vi "PUT File.vi"(6 "timeout (10000)":i32=10000, 7 "output file":path=path "", 8 "error in (no error)":errorcluster, 9 "file":path, 10 "url":string, 11 "HTTP Client Advanced in":refnum<class "HTTP Client Advanced.lvclass">) -> (0 "error out":errorcluster, 1 "body":string, 2 "headers":string, 3 "HTTP Client Advanced out":refnum<class "HTTP Client Advanced.lvclass">)   [LabVIEW 2021, in "HTTP Client Advanced.lvclass"]
uses:
  HTTP Client Advanced.lvclass
  HTTP Client Advanced.lvclass/HTTP Client Advanced.ctl
  <vilib>/NI/Advanced HTTP Client/Session.lvclass
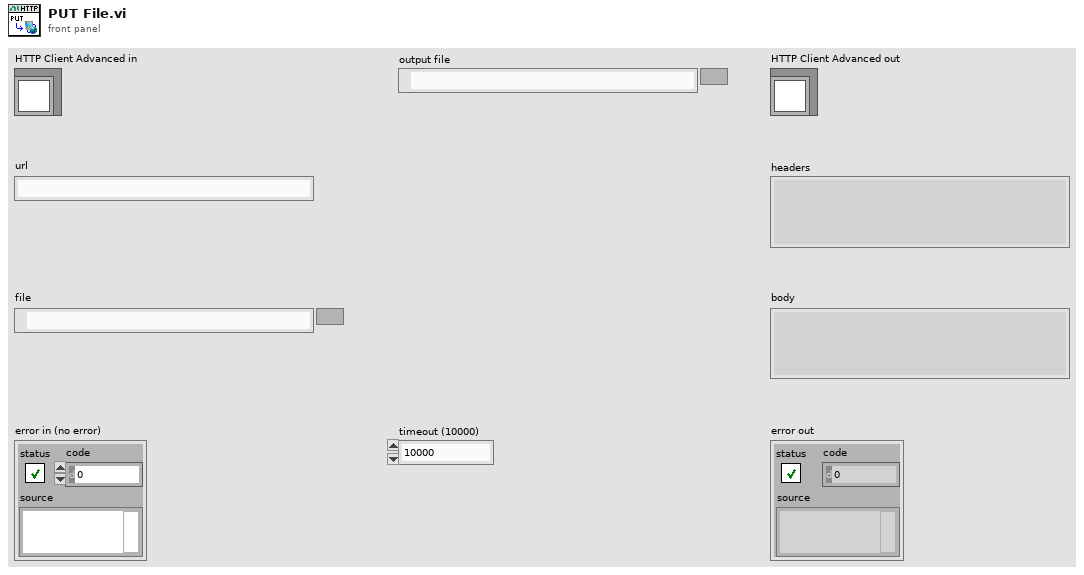
[diagram p1: front panel]
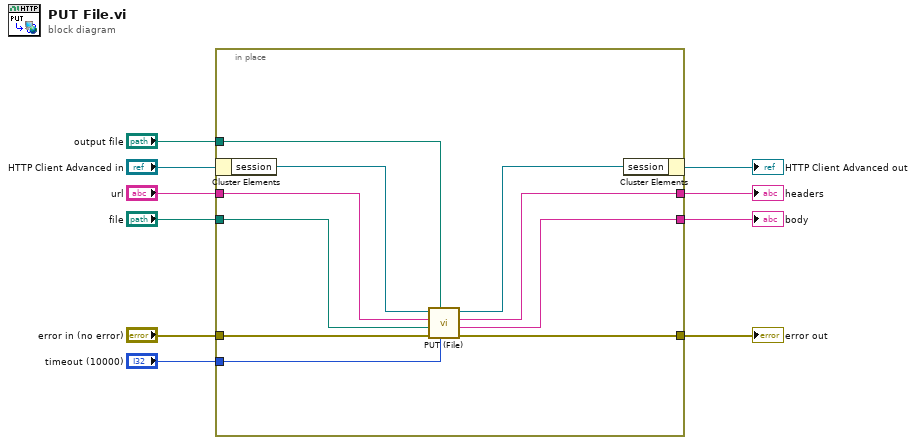
[diagram p0: block diagram]
diagram:
  n1 = in-place {
    in-place-border: "error in (no error)" -> [w20]
    in-place-border: [w19] -> w8
    in-place-border: "output file" -> [w16]
    in-place-border: "url" -> [w15]
    in-place-border: "file" -> [w14]
    in-place-border: "timeout (10000)" -> [w13]
    in-place-border: [w12] -> w2
    in-place-border: [w11] -> w1
    n2 = in-place-cluster #1("HTTP Client Advanced in") -> ("session"=w18:refnum<class "Session.lvclass">)
    n3 = call <vilib>:"PUT (File).vi"("timeout"=w13, "output file"=w16, "error in"=w20, "file"=w14, "url"=w15, "session in"=w18) -> ("error out"=w19:errorcluster, "body"=w11:string, "headers"=w12:string, "session out"=w17:refnum<class "Session.lvclass">)  [unwired: 1 in, 1 out]
    n4 = in-place-cluster #1("session"=w17) -> (→"HTTP Client Advanced out":refnum<class "HTTP Client Advanced.lvclass">)
  }
  "error out" <- w8
  "headers" <- w2
  "body" <- w1
